vi "Inner Join.vi"() -> ()   [LabVIEW 2020]
uses:
  a75eeadb-a20a-426b-b48b-c9c06ab4b909.vi
panel:
  out "array with duplicates removed":string[][](array[string])
  in  "Array 2":string[][](array[string])
  in  "Array":string[][](array[string])
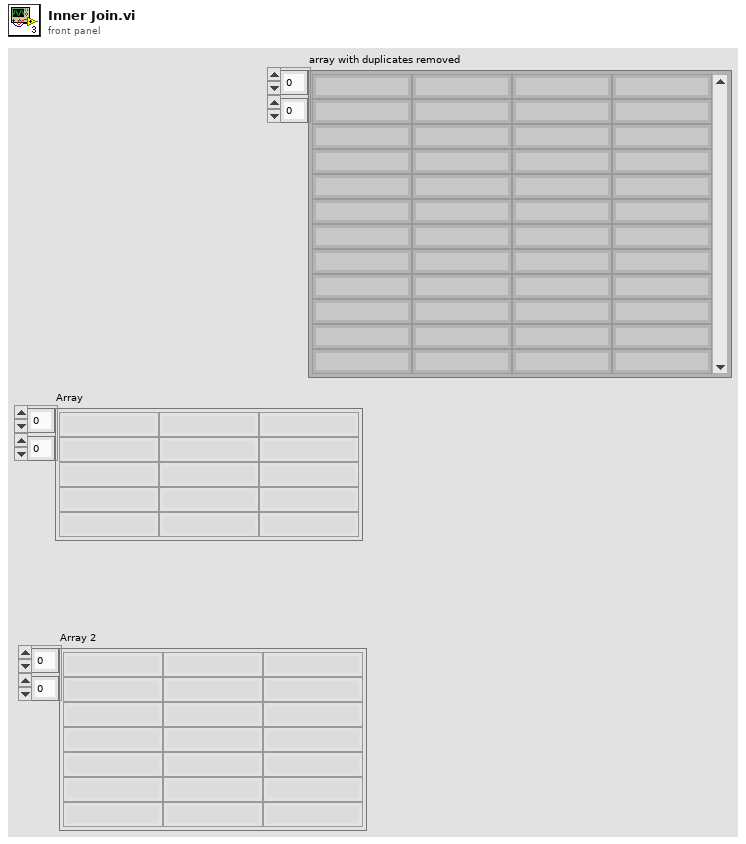
[diagram p1: front panel]
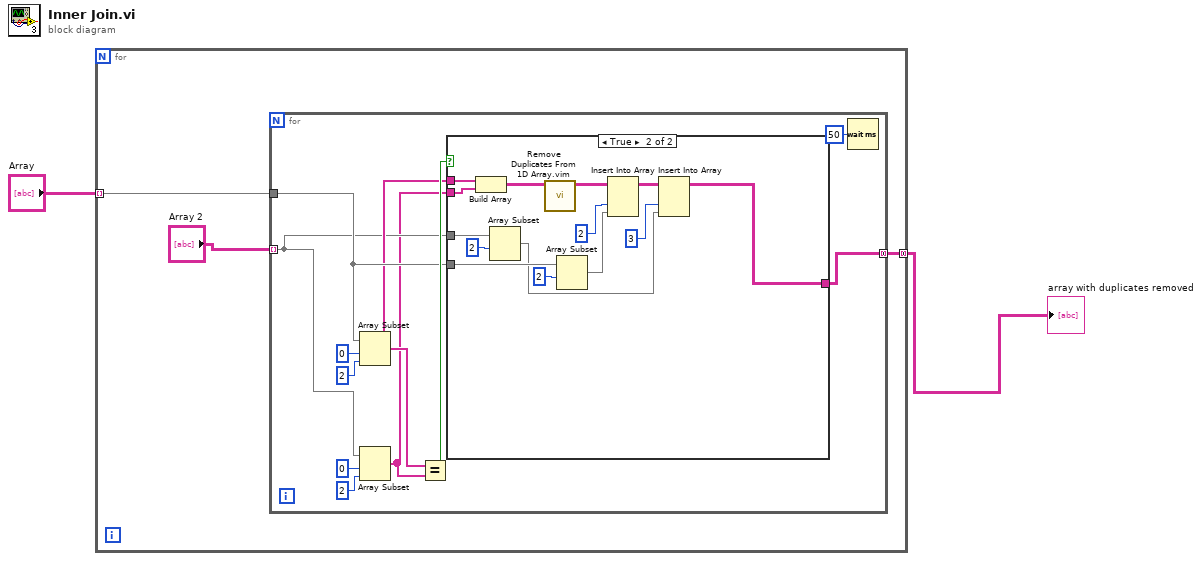
[diagram p0: block diagram]
diagram:
  n1 = for {
    tunnel: "Array" -> [w4] mode=indexing
    tunnel: [w3] -> w1 mode=concatenating
    n2 = for {
      tunnel: "Array 2" -> [w8] mode=indexing
      tunnel: w4 -> [w10]
      tunnel: [w15] -> w3 mode=concatenating
      n3 = Array Subset(array=w10, index=0, length=2) -> (w9:string[])
      n4 = Array Subset(array=w8, index=0, length=2) -> (w7:string[])
      n5 = Equal?(x=w9, y=w7) -> (x = y?=w16:bool)
      n6 = case shown="True" w16 {
        tunnel: [_ w19] -> w15
        tunnel: w10 -> [_ w26]
        tunnel: w8 -> [_ w23]
        tunnel: w9 -> [_ w30]
        tunnel: w7 -> [_ w29]
        frame False {
        }
        frame True {
          n7 = Build Array(w30, w29) -> (w28:string[][])
          n8 = Array Subset(array=w23, index=2) -> (w20:string[])  [unwired: 1 in]
          n9 = call "Remove Duplicates From 1D Array.vim"("array"=w28) -> ("array with duplicates removed"=w27:string[][])  [unwired: 10 in]
          n10 = Array Subset(array=w26, index=2) -> (w25:string[])  [unwired: 1 in]
          n11 = Insert Into Array(array=w27, index (col)=2 ("index (row)"), new element=w25) -> (w21:string[][])  [unwired: 1 in]
          n12 = Insert Into Array(array=w21, index (col)=3 ("index (row)"), new element=w20) -> (w19:string[][])  [unwired: 1 in]
        }
      }
      n13 = Wait (ms)(milliseconds to wait=u32 50) -> ()  [unwired: 1 out]
    }
  }
  "array with duplicates removed" <- w1
